vi "SLSC_12201_AsynRTEngine.vi"(10 "Parameters":variant, 11 "Process":refnum<class "Process.lvclass">) -> ()   [LabVIEW 2020, in "SLSC-12201 DIO Engine.lvlib"]
uses:
  SLSC-12201 DIO Engine.lvlib
  <vilib>/NI/NIVS Inline Async API/_VS Inline Async API/Process/Process.lvclass
  Types/Async Engine State Control.ctl
  <vilib>/NI/NIVS Inline Async API/_VS Inline Async API/Process/Process.lvclass/Process.ctl
  Shared/Compiled.Settings
  Shared/SLSC Dynamic Channel.ctl
  Shared/SLSC Dynamic Channel Type.ctl
  <vilib>/NI/NIVS Inline Async API/_Data Access Engine/Access Type Classes/Read/Read.lvclass/Read.ctl
  <vilib>/NI/NIVS Inline Async API/_Data Access Engine/Access Type Classes/ReadWrite/ReadWrite.lvclass/ReadWrite.ctl
  <vilib>/NI/NIVS Inline Async API/_Data Access Engine/Access Type Classes/Write/Write.lvclass/Write.ctl
  <vilib>/NI/NIVS Inline Async API/_Data Access Engine/Data Access Engine/Methods/Read.Data.vi
  <vilib>/NI/NIVS Inline Async API/_Data Access Engine/Data Access Engine/Methods/Read.Data.Detect.vi
  <vilib>/NI/NIVS Inline Async API/_Data Access Engine/Data Access Engine/Methods/Write.Data.vi
  <vilib>/NI/NIVS Inline Async API/_Data Access Engine/Data Access Engine/Methods/ReadWrite.Data.vi
  <vilib>/NI/NIVS Inline Async API/_VS Inline Async API/Process/Data Member Access/Read Data Access.vi
  <vilib>/NI/NIVS Inline Async API/_VS Inline Async API/Error Handling Process/SubVIs/Error.ConvertArray.vi
  SLSC_Determine_Resource.vi
  <vilib>/NI/NIVS Inline Async API/_Data Access Engine/Access Type Classes/Read/Read.ProcessData.vi
  <vilib>/NI/NIVS Inline Async API/_Data Access Engine/Access Type Classes/Read/Read.ProcessData.Detect.vi
  <vilib>/NI/NIVS Inline Async API/_Data Access Engine/Access Type Classes/Write/Write.ProcessData.vi
  <vilib>/NI/NIVS Inline Async API/_Data Access Engine/Access Type Classes/ReadWrite/ReadWrite.ProcessData.vi
  <vilib>/NI/NIVS Inline Async API/_Data Access Engine/Access Type Classes/Write/Write.Buffer.vi
  <vilib>/NI/NIVS Inline Async API/_Data Access Engine/Access Type Classes/Write/Write.Commit.vi
  Shared/Constants.vi
  <vilib>/NI/NIVS Inline Async API/_Data Access Engine/Data Access Engine/Methods/Read.Lookup.vi
  <vilib>/NI/NIVS Inline Async API/_Data Access Engine/Data Access Engine/Methods/ReadWrite.Lookup.vi
  <vilib>/NI/NIVS Inline Async API/_Data Access Engine/Data Access Engine/Methods/Write.Lookup.vi
  <vilib>/SLSC/Set Generic Property.vi
  <vilib>/SLSC/Set Generic Property (Bool).vi
  <vilib>/SLSC/Set Generic Property (DBL).vi
  <vilib>/SLSC/Set Generic Property (I32).vi
  <vilib>/SLSC/Set Generic Property (I64).vi
  <vilib>/SLSC/Set Generic Property (String).vi
  <vilib>/SLSC/Set Generic Property (U32).vi
  <vilib>/SLSC/Set Generic Property (U64).vi
  <vilib>/SLSC/Commit Properties.vi
  <vilib>/SLSC/Commit Properties for Devices.vi
  <vilib>/SLSC/Execute Command.vi
  <vilib>/SLSC/Execute Device Command.vi
  <vilib>/SLSC/Execute Phys Chan Command.vi
  <vilib>/SLSC/Get Generic Property.vi
  <vilib>/SLSC/Get Generic Property (Bool).vi
  <vilib>/SLSC/Get Generic Property (DBL).vi
  <vilib>/SLSC/Get Generic Property (I32).vi
  <vilib>/SLSC/Get Generic Property (I64).vi
  <vilib>/SLSC/Get Generic Property (String).vi
  <vilib>/SLSC/Get Generic Property (U32).vi
  <vilib>/SLSC/Get Generic Property (U64).vi
  <vilib>/SLSC/Close Session.vi
  <vilib>/NI/NIVS Inline Async API/_Data Access Engine/Data Access Engine/Data Access Engine.lvclass
  <vilib>/NI VeriStand/Custom Device Tools/Custom Device Utility Library/Custom Device Utility Library.lvlib
  <vilib>/SLSC/SLSC.lvlib
  Shared/SLSC-12201 DIO Shared.lvlib
  <vilib>/NI/NIVS Inline Async API/_Data Access Engine/Access Type Classes/Write/Write.lvclass
panel:
  out "Async Engine Control":T1
  out "error IO":errorcluster
  in  "LoopRate(ms)":u32=500
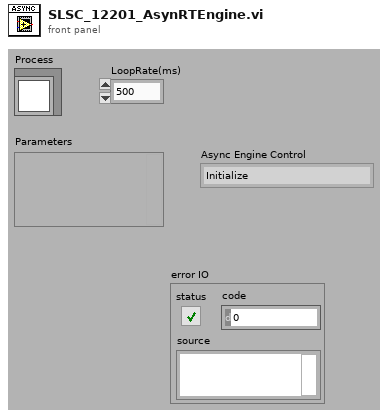
[diagram p1: front panel]
types:
  T1 = typedef "SLSC-12201 DIO Engine.lvlib/Async Engine State Control.ctl" = enum16{"Initialize", "Configure", "Run", "Reset", "Shutdown"}
  T2 = typedef "SLSC-12201 DIO Shared.lvlib/Compiled.Settings" = cluster{"Name":string, "SLSC IP -Module Name":string, "Slot #":i32, "Configuration Data":cluster{"Properties":cluster{"Boolean Properties":cluster{"property":refnum<k21>, "Value":bool, "SLSC Item":refnum<k21>}[], "Double Properties":cluster{"property":refnum<k21>, "Double Write":dbl, "SLSC Item":refnum<k21>}[], "I32 Properties":cluster{"property":refnum<k21>, "Int32 Write":i32, "SLSC Item":refnum<k21>}[], "I64 Properties":cluster{"property":refnum<k21>, "Int64 Write":i64, "SLSC Item":refnum<k21>}[], "String Properties":cluster{"property":refnum<k21>, "String Write":string, "SLSC Item":refnum<k21>}[], "U32 Properties":cluster{"property":refnum<k21>, "UInt32 Write":u32, "SLSC Item":refnum<k21>}[], "U64 Properties":cluster{"property":refnum<k21>, "UInt64 Write":u64, "SLSC Item":refnum<k21>}[]}}, "SLSC Set Properties":T3[], "SLSC Get Properties":T3[], "SLSC Commands":T3[], "Username":string, "Password":string, "Support Modules":cluster{"Dev.ProductNumber":u32, "Dev.VendorNumber":u32}[]}
  T3 = typedef "SLSC-12201 DIO Shared.lvlib/SLSC Dynamic Channel.ctl" = cluster{"SLSC Item":string, "property":string, "Data Type":T4, "Value":variant}
  T4 = typedef "SLSC-12201 DIO Shared.lvlib/SLSC Dynamic Channel Type.ctl" = enum16{"Bool", "Double", "I32", "I64", "String", "U32", "U64", "EnumI32"}
  T5 = typedef "Data Access Engine.lvlib/Data Access Engine.lvclass/Read.DVR.ctl" = refnum<data-value>
  T6 = typedef "Data Access Engine.lvlib/Data Access Engine.lvclass/ReadWrite.DVR.ctl" = refnum<data-value>
  T7 = typedef "Data Access Engine.lvlib/Data Access Engine.lvclass/Write.DVR.ctl" = refnum<data-value>
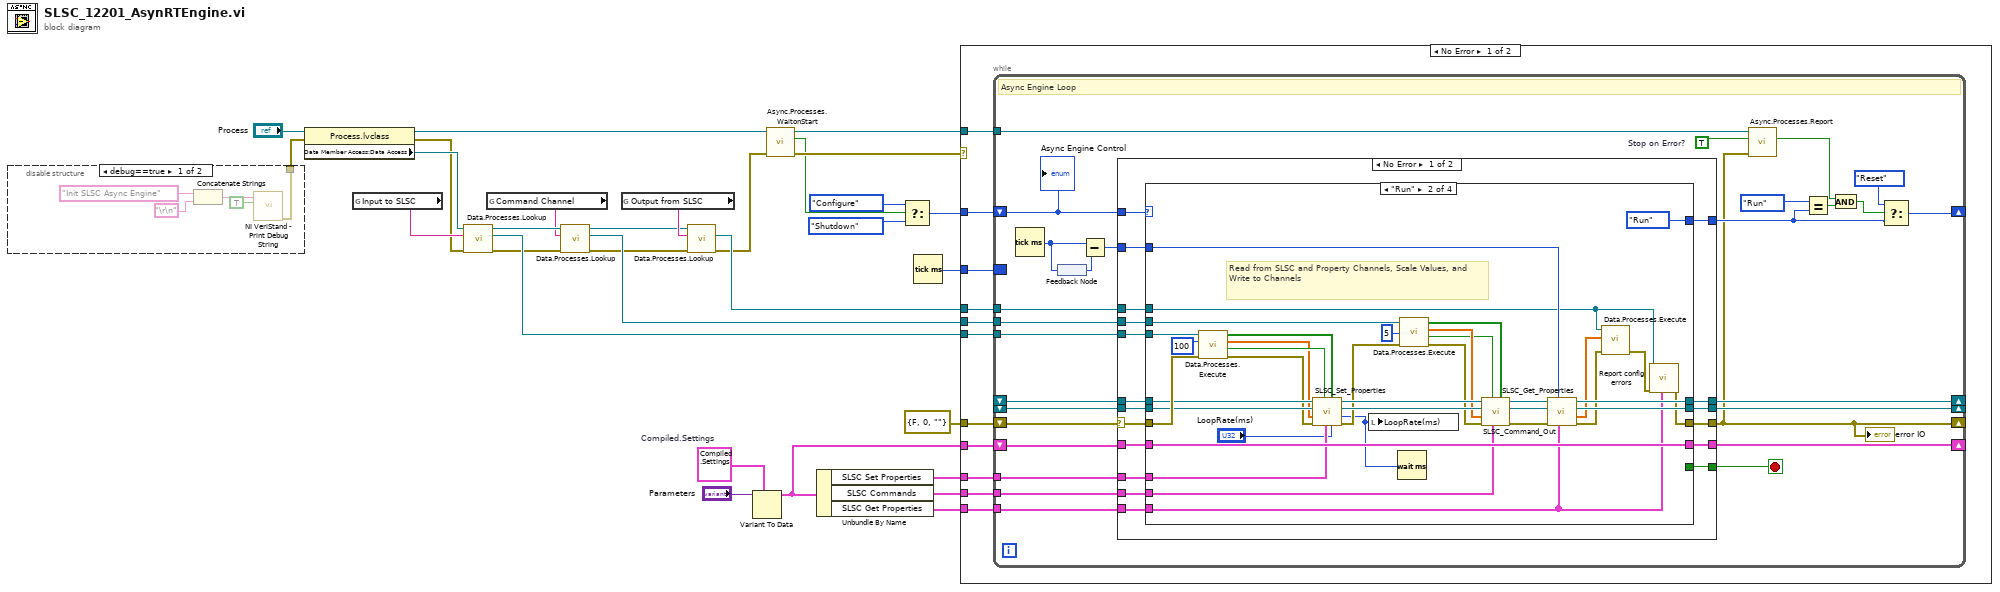
[diagram p0: block diagram]
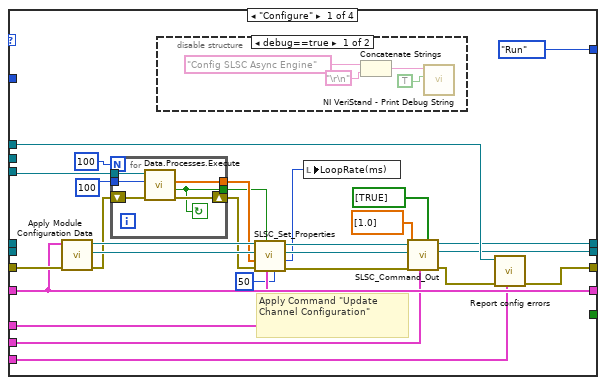
[diagram p3: hidden frame]
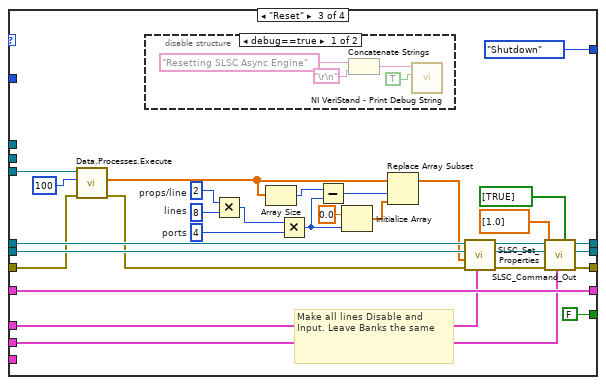
[diagram p5: hidden frame]
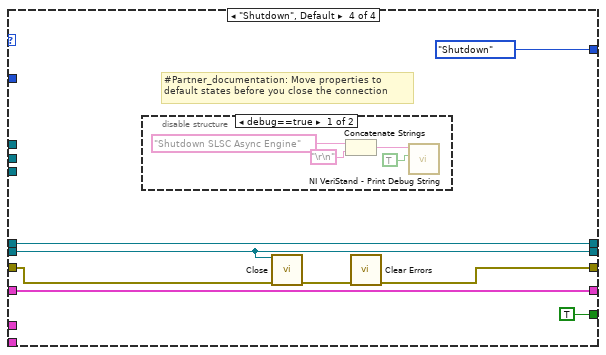
[diagram p7: hidden frame]
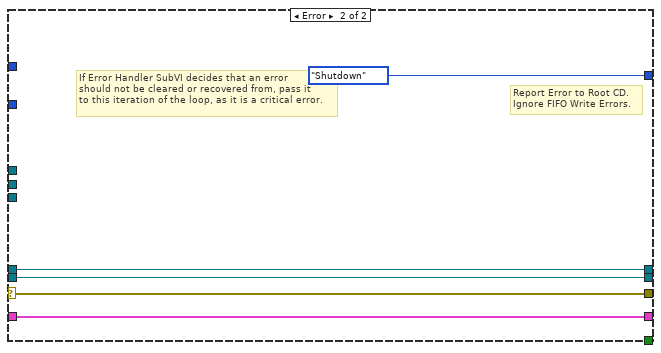
[diagram p9: hidden frame]
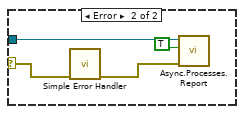
[diagram p10: hidden frame]
diagram:
  w23 = T2 {"Name"="", "SLSC IP -Module Name"="", "Slot #"=0, "Configuration Data"={"Properties"={"Boolean Properties"=[], "Double Properties"=[], "I32 Properties"=[], "I64 Properties"=[], "String Properties"=[], "U32 Properties"=[], "U64 Properties"=[]}}, "SLSC Set Properties"=[], "SLSC Get Properties"=[], "SLSC Commands"=[], "Username"="", "Password"="", "Support Modules"=[]}  # Compiled.Settings
  n1 = disable-structure shown="debug==true" {
    disable-tunnel: [w31 _] -> w13
    frame condition #0 {
      n2 = Concatenate Strings("Init SLSC Async Engine" ("Message"), "\r\n") -> (w34:string)
      n3 = call <vilib>:"NI VeriStand - Print Debug String.vi"("Add to log file? (F)"=TRUE ("Add to log file? (T)"), "Message"=w34) -> ("error out"=w31:errorcluster)  [unwired: 9 in]
    }
    frame condition #1 (active) {
    }
  }
  n4 = property class="Process.lvclass"(reference="Process", error in=w13) -> (reference out=w25:refnum<class "Process.lvclass">, error out=w2:errorcluster, "Data Member Access:Data Access"=w3:refnum<class "Data Access Engine.lvclass">)
  n5 = global read "Constants.vi" "Input to SLSC"() -> (w15:string)
  n6 = call-poly <vilib>:"Data.Processes.Lookup.vi"("error in (no error)"=w2, "Name"=w15, "Data Access API in"=w3) -> ("error out"=w10:errorcluster, "Ref"=w28:T5, "Data Access API out"=w11:refnum<class "Data Access Engine.lvclass">)  [unwired: 5 in, 1 out]
  n7 = global read "Constants.vi" "Command Channel"() -> (w9:string)
  n8 = call-poly <vilib>:"Data.Processes.Lookup.vi"("error in (no error)"=w10, "Name"=w9, "Data Access API in"=w11) -> ("error out"=w5:errorcluster, "Ref"=w8:T6, "Data Access API out"=w4:refnum<class "Data Access Engine.lvclass">)  [unwired: 5 in, 1 out]
  n9 = global read "Constants.vi" "Output from SLSC"() -> (w16:string)
  n10 = call-poly <vilib>:"Data.Processes.Lookup.vi"("error in (no error)"=w5, "Name"=w16, "Data Access API in"=w4) -> ("error out"=w1:errorcluster, "Ref"=w27:T7)  [unwired: 5 in, 2 out]
  n11 = Variant To Data(type=w23, Variant="Parameters") -> (data=w18:T2)  [unwired: 1 in, 1 out]
  n12 = call <vilib>:"Async.Processes.WaitonStart.vi"("error in (no error)"=w1, "Process"=w25) -> ("error out"=w29:errorcluster, "Execute"=w22:bool, "Process out"=w30:refnum<class "Process.lvclass">)  [unwired: 7 in]
  n13 = Unbundle By Name(w18) -> ("SLSC Set Properties"=w17:T3[], "SLSC Commands"=w12:T3[], "SLSC Get Properties"=w6:T3[])
  n14 = Select(t=Async_Engine_State_Control."Configure", s=w22, f=Async_Engine_State_Control."Shutdown") -> (s? t:f=w19:T1)
  n15 = Tick Count (ms)() -> (millisecond timer value=w14:u32)
  n16 = case shown="No Error" w29 {
    selector: w29 -> [_ w219]
    tunnel: w30 -> [w46 w220]
    tunnel: w27 -> [w45 _]
    tunnel: w28 -> [w44 _]
    tunnel: w18 -> [w39 _]
    tunnel: errorcluster {"status"=FALSE, "code"=0, "source"=""} ("error constant") -> [w43 _]
    tunnel: w19 -> [w42 _]
    tunnel: w17 -> [w41 _]
    tunnel: w14 -> [w40 _]
    tunnel: w12 -> [w38 _]
    tunnel: w8 -> [w37 _]
    tunnel: w6 -> [w36 _]
    frame No Error {
      n17 = while {
        shift-right: [w47] -> _
        shift-left: w43 -> [w74]
        shift-right: [w48] -> _
        shift-left: w42 -> [w73]
        shift-right: [w72] -> _
        shift-left: w39 -> [w71]
        shift-right: [w70] -> _
        shift-left: _ -> [w69]
        tunnel: w44 -> [w68]
        tunnel: w45 -> [w67]
        tunnel: w46 -> [w66]
        tunnel: w41 -> [w65]
        shift-right: [w64] -> _
        shift-left: _ -> [w63]
        border: w40 -> [_]
        tunnel: w38 -> [w55]
        tunnel: w37 -> [w54]
        tunnel: w36 -> [w53]
        stop <- w58 stop-if-true
        w62 = TRUE  # Stop on Error?
        # "Async Engine Loop"
        n18 = Tick Count (ms)() -> (millisecond timer value=w61:u32)
        n19 = feedback-in #1(w61) -> ()
        n20 = feedback #1() -> (w60:u32)
        n21 = Subtract(x=w61, y=w60) -> (x-y=w59:u32)
        n22 = case shown="No Error" w74 {
          selector: w74 -> [w91 w213]
          tunnel: [w84 w213] -> w47
          tunnel: w73 -> [w92 _]
          tunnel: [w85 Async_Engine_State_Control."Shutdown"] -> w49
          tunnel: [w90 _] -> w58
          tunnel: [w89 w216] -> w72
          tunnel: w71 -> [w88 w216]
          tunnel: [w87 w215] -> w70
          tunnel: w69 -> [w86 w215]
          tunnel: w68 -> [w83 _]
          tunnel: w67 -> [w82 _]
          tunnel: w65 -> [w81 _]
          tunnel: [w80 w212] -> w64
          tunnel: w63 -> [w79 w212]
          tunnel: w59 -> [w78 _]
          tunnel: w55 -> [w77 _]
          tunnel: w54 -> [w76 _]
          tunnel: w53 -> [w75 _]
          frame No Error {
            n23 = case shown="\"Run\"" w92 {
              tunnel: w91 -> [w119 w162 w177 w200]
              tunnel: [w116 w133 w168 w203] -> w84
              tunnel: [Async_Engine_State_Control."Run" Async_Engine_State_Control."Run" Async_Engine_State_Control."Shutdown" Async_Engine_State_Control."Shutdown"] -> w85
              tunnel: [_ _ FALSE TRUE] -> w90
              tunnel: [w115 w165 w194 w206] -> w89
              tunnel: w88 -> [w115 w165 w194 w206]
              tunnel: [w113 w156 w169 w201] -> w87
              tunnel: w86 -> [_ w160 w188 w201]
              tunnel: w83 -> [w106 w163 w191 _]
              tunnel: w82 -> [w117 w134 _ _]
              tunnel: w81 -> [w102 w159 w190 _]
              tunnel: [w114 w157 w170 w202] -> w80
              tunnel: w79 -> [_ w158 w189 w202]
              tunnel: w78 -> [_ w154 _ _]
              tunnel: w77 -> [w96 w144 w167 _]
              tunnel: w76 -> [_ w152 _ _]
              tunnel: w75 -> [w109 w132 _ _]
              frame "Configure" {
                # "Apply Command \"Update Channel Configuration\""
                n24 = call "Apply Module Configuration Data.vi"("Error In"=w119, "Compiled.Settings"=w115) -> ("Error Out"=w101:errorcluster, "Device Session"=w107:refnum<k21>, "SLSC Module Name"=w108:refnum<k21>)  [unwired: 7 in]
                n25 = for {
                  N: 100 -> [_]
                  tunnel: w106 -> [w125]
                  tunnel: [w124] -> w105
                  tunnel: 100 ("timeout ms") -> [w123]
                  tunnel: [w120] -> w103
                  shift-right: [w121] -> w100
                  shift-left: w101 -> [w122]
                  stop <- w120 continue-if-true
                  n26 = call-poly <vilib>:"Data.Processes.Execute.vi"("error in (no error)"=w122, "timeout ms"=w123, "Ref"=w125) -> ("error out"=w121:errorcluster, "Timeout?"=w120:bool, "Values"=w124:dbl[])  [unwired: 6 in]
                }
                n27 = disable-structure shown="debug==true" {
                  frame condition #0 {
                    n28 = Concatenate Strings("Config SLSC Async Engine" ("Message"), "\r\n") -> (w127:string)
                    n29 = call <vilib>:"NI VeriStand - Print Debug String.vi"("Add to log file? (F)"=TRUE ("Add to log file? (T)"), "Message"=w127) -> ()  [unwired: 9 in, 1 out]
                  }
                  frame condition #1 (active) {
                  }
                }
                n30 = call "SLSC_Set_Properties.vi"("LoopRate(ms) in"=u32 50, "SLSC Dynamic Outputs"=w102, "Stop Updating?"=w103, "error in"=w100, "Values"=w105, "session in"=w107, "SLSC Module Name"=w108) -> ("error out"=w97:errorcluster, "LoopRate(ms)"=w94:u32, "session out"=w98:refnum<k21>, "SLSC Module Name"=w99:refnum<k21>)  [unwired: 1 in]
                n31 = local write "LoopRate(ms)"(w94) -> ()
                n32 = call "SLSC_Command_Out.vi"("Detect?"=bool[] [TRUE], "SLSC Dynamic Commands"=w96, "error in"=w97, "Values"=dbl[] [1.0], "session in"=w98, "SLSC Module Name"=w99) -> ("error out"=w110:errorcluster, "session out"=w113:refnum<k21>, "SLSC Module Name"=w114:refnum<k21>)  [unwired: 3 in]
                n33 = call "Report config errors.vi"("SLSC Dynamic Inputs"=w109, "error in (no error)"=w110, "Data Value Reference in"=w117) -> ("error out"=w116:errorcluster)  [unwired: 8 in]
              }
              frame "Run" {
                # "Read from SLSC and Property Channels, Scale Values, and Write to Channels"
                n34 = call-poly <vilib>:"Data.Processes.Execute.vi"("error in (no error)"=w162, "timeout ms"=100, "Ref"=w163) -> ("error out"=w143:errorcluster, "Timeout?"=w140:bool, "Values"=w137:dbl[], "Detect?"=w136:bool[])  [unwired: 5 in]
                n35 = call "SLSC_Set_Properties.vi"("LoopRate(ms) in"="LoopRate(ms)", "Detect?"=w136, "SLSC Dynamic Outputs"=w159, "Stop Updating?"=w140, "error in"=w143, "Values"=w137, "session in"=w160, "SLSC Module Name"=w158) -> ("error out"=w142:errorcluster, "LoopRate(ms)"=w130:u32, "session out"=w149:refnum<k21>, "SLSC Module Name"=w150:refnum<k21>)
                n36 = local write "LoopRate(ms)"(w130) -> ()
                n37 = Wait (ms)(milliseconds to wait=w130) -> ()  [unwired: 1 out]
                n38 = call-poly <vilib>:"Data.Processes.Execute.vi"("error in (no error)"=w142, "timeout ms"=5, "Ref"=w152) -> ("error out"=w141:errorcluster, "Timeout?"=w139:bool, "Data"=w146:dbl[], "Detect?"=w138:bool[])  [unwired: 5 in]
                n39 = call "SLSC_Command_Out.vi"("Detect?"=w138, "SLSC Dynamic Commands"=w144, "Timeout?"=w139, "error in"=w141, "Values"=w146, "session in"=w149, "SLSC Module Name"=w150) -> ("error out"=w145:errorcluster, "session out"=w147:refnum<k21>, "SLSC Module Name"=w148:refnum<k21>)  [unwired: 2 in]
                n40 = call "SLSC_Get_Properties.vi"("SLSC Dynamic Inputs"=w132, "LoopDuration(ms)"=w154, "error in"=w145, "session in"=w147, "SLSC Module Name"=w148) -> ("error out"=w155:errorcluster, "Values"=w153:dbl[], "session out"=w156:refnum<k21>, "SLSC Module Name"=w157:refnum<k21>)  [unwired: 3 in]
                n41 = call-poly <vilib>:"Data.Processes.Execute.vi"("error in (no error)"=w155, "Values"=w153, "Ref"=w134) -> ("error out"=w135:errorcluster)  [unwired: 8 in]
                n42 = call "Report config errors.vi"("SLSC Dynamic Inputs"=w132, "error in (no error)"=w135, "Data Value Reference in"=w134) -> ("error out"=w133:errorcluster)  [unwired: 8 in]
              }
              frame "Reset" {
                w181 = 4  # ports
                w183 = 8  # lines
                w184 = 2  # props/line
                # "Make all lines Disable and Input. Leave Banks the same"
                n43 = call-poly <vilib>:"Data.Processes.Execute.vi"("error in (no error)"=w177, "timeout ms"=100, "Ref"=w191) -> ("error out"=w176:errorcluster, "Values"=w180:dbl[])  [unwired: 6 in, 1 out]
                n44 = disable-structure shown="debug==true" {
                  frame condition #0 {
                    n45 = Concatenate Strings("Resetting SLSC Async Engine" ("Message"), "\r\n") -> (w197:string)
                    n46 = call <vilib>:"NI VeriStand - Print Debug String.vi"("Add to log file? (F)"=TRUE ("Add to log file? (T)"), "Message"=w197) -> ()  [unwired: 9 in, 1 out]
                  }
                  frame condition #1 (active) {
                  }
                }
                n47 = Multiply(x=w184, y=w183) -> (x*y=w182:i32)
                n48 = Array Size(array=w180) -> (size(s)=w179:i32)
                n49 = Multiply(x=w182, y=w181) -> (x*y=w178:i32)
                n50 = Subtract(x=w179, y=w178) -> (x-y=w166:i32)
                n51 = Initialize Array(0.0 ("Default value"), w178) -> (w186:dbl[])
                n52 = Replace Array Subset(array=w180, new element=w186, index=w166) -> (w185:dbl[])
                n53 = call "SLSC_Set_Properties.vi"("SLSC Dynamic Outputs"=w190, "error in"=w176, "Values"=w185, "session in"=w188, "SLSC Module Name"=w189) -> ("error out"=w171:errorcluster, "session out"=w172:refnum<k21>, "SLSC Module Name"=w173:refnum<k21>)  [unwired: 3 in, 1 out]
                n54 = call "SLSC_Command_Out.vi"("Detect?"=bool[] [TRUE], "SLSC Dynamic Commands"=w167, "error in"=w171, "Values"=dbl[] [1.0], "session in"=w172, "SLSC Module Name"=w173) -> ("error out"=w168:errorcluster, "session out"=w169:refnum<k21>, "SLSC Module Name"=w170:refnum<k21>)  [unwired: 3 in]
              }
              frame "Shutdown", Default {
                # "#Partner_documentation: Move properties to \ndefault states before you close the connection"
                n55 = disable-structure shown="debug==true" {
                  frame condition #0 {
                    n56 = Concatenate Strings("Shutdown SLSC Async Engine" ("Message"), "\r\n") -> (w209:string)
                    n57 = call <vilib>:"NI VeriStand - Print Debug String.vi"("Add to log file? (F)"=TRUE ("Add to log file? (T)"), "Message"=w209) -> ()  [unwired: 9 in, 1 out]
                  }
                  frame condition #1 (active) {
                  }
                }
                n58 = call-poly <vilib>:"Close.vi"("session in"=w201, "error in (no error)"=w200) -> ("error out"=w204:errorcluster)  [unwired: 13 in]
                n59 = call <vilib>:"Clear Errors.vi"("error in (no error)"=w204) -> ("error out"=w203:errorcluster)  [unwired: 5 in, 1 out]
              }
            }
          }
          frame Error {
            # "If Error Handler SubVI decides that an error\nshould not be cleared or recovered from, pass it\nto this iteration of the loop, as it is a critical error."
            # "Report Error to Root CD.\nIgnore FIFO Write Errors."
          }
        }
        "error IO" <- w47
        n60 = call <vilib>:"Async.Processes.Report.vi"("Error"=w47, "Stop Async on Error?"=w62, "Process in"=w66) -> ("Stop"=w57:bool)  [unwired: 7 in, 1 out]
        n61 = Equal?(x=Async_Engine_State_Control."Run", y=w49) -> (x = y?=w51:bool)
        n62 = And(x=w57, y=w51) -> (x .and. y?=w52:bool)
        n63 = Select(t=Async_Engine_State_Control."Reset", s=w52, f=w49) -> (s? t:f=w48:T1)
        "Async Engine Control" <- w73
      }
    }
    frame Error {
      n64 = call <vilib>:"Simple Error Handler.vi"("error in (no error)"=w219) -> ("error out"=w217:errorcluster)  [unwired: 4 in, 4 out]
      n65 = call <vilib>:"Async.Processes.Report.vi"("Error"=w217, "Stop Async on Error?"=TRUE ("Stop on Error?"), "Process in"=w220) -> ()  [unwired: 7 in, 2 out]
    }
  }
